vi "Save Scores.vi"(8 "error in (no error)":errorcluster, 9 "Test Summary":string, 10 "Score":T1, 11 "LLB Path":path) -> ()   [LabVIEW 2020, in "SOL-Scorer.lvlib"]
uses:
  SOL-Scorer.lvlib
  SoL Scoring/Score.ctl
  SoL Scoring/Score Entry.ctl
  <vilib>/Utility/config.llb/Write Key (Double).vi
  <vilib>/Utility/config.llb/Write Key (String).vi
  <vilib>/Utility/config.llb/Write Key (I32).vi
  <vilib>/Utility/config.llb/NI_LVConfig.lvlib
  SoL Scoring/SoL Scoring.lvlib
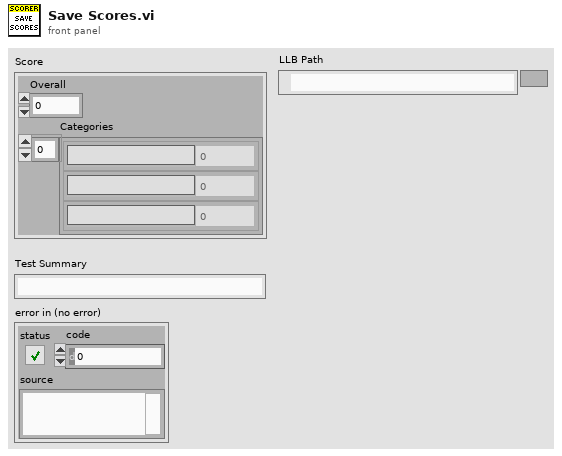
[diagram p1: front panel]
types:
  T1 = typedef "SoL Scoring.lvlib/Score.ctl" = cluster{"Overall":dbl, "Categories":T2[]}
  T2 = typedef "SoL Scoring.lvlib/Score Entry.ctl" = cluster{"Category":string, "Value":dbl}
  T3 = typedef "NI_LVConfig.lvlib/Config Data RefNum.ctl" = refnum<k1>
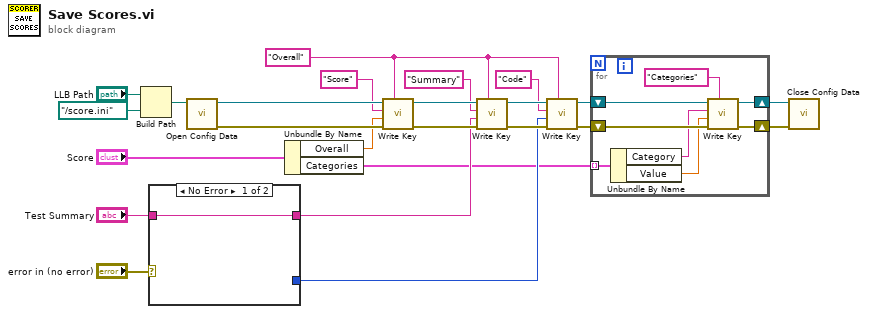
[diagram p0: block diagram]
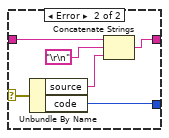
[diagram p2: hidden frame]
diagram:
  w8 = "Overall" ("section")
  n1 = Build Path(base path="LLB Path", name or relative path=path "../score.ini") -> (appended path=w22:path)
  n2 = case shown="No Error" "error in (no error)" {
    selector: "error in (no error)" -> [_ w29]
    tunnel: "Test Summary" -> [w25 w31]
    tunnel: [w25 w27] -> w11
    tunnel: [_ w26] -> w6
    frame No Error {
    }
    frame Error {
      n3 = Unbundle By Name(w29) -> ("source"=w28:string, "code"=w26:i32)
      n4 = Concatenate Strings(w31, "\r\n", w28) -> (w27:string)
    }
  }
  n5 = call <vilib>:"Open Config Data.vi"("configuration file path"=w22) -> ("error out"=w15:errorcluster, "refnum"=w19:T3)  [unwired: 8 in, 1 out]
  n6 = Unbundle By Name("Score") -> ("Overall"=w13:dbl, "Categories"=w3:T2[])
  n7 = call-poly <vilib>:"Write Key.vi"("section"=w8, "error in (no error)"=w15, "value"=w13, "key"="Score", "refnum"=w19) -> ("error out"=w14:errorcluster, "refnum out"=w17:T3)  [unwired: 4 in, 1 out]
  n8 = call-poly <vilib>:"Write Key.vi"("section"=w8, "error in (no error)"=w14, "value"=w11, "key"="Summary", "refnum"=w17) -> ("error out"=w9:errorcluster, "refnum out"=w10:T3)  [unwired: 4 in, 1 out]
  n9 = call-poly <vilib>:"Write Key.vi"("section"=w8, "error in (no error)"=w9, "value"=w6, "key"="Code", "refnum"=w10) -> ("error out"=w4:errorcluster, "refnum out"=w5:T3)  [unwired: 4 in, 1 out]
  n10 = for {
    shift-right: [w33] -> w2
    shift-left: w5 -> [w39]
    shift-right: [w32] -> w1
    shift-left: w4 -> [w37]
    tunnel: w3 -> [w36] mode=indexing
    n11 = Unbundle By Name(w36) -> ("Category"=w35:string, "Value"=w34:dbl)
    n12 = call-poly <vilib>:"Write Key.vi"("section"="Categories", "error in (no error)"=w37, "value"=w34, "key"=w35, "refnum"=w39) -> ("error out"=w32:errorcluster, "refnum out"=w33:T3)  [unwired: 4 in, 1 out]
  }
  n13 = call <vilib>:"Close Config Data.vi"("error in (no error)"=w1, "refnum"=w2) -> ()  [unwired: 8 in, 2 out]
